vi "Teleop.vi"(10 "Match Info":T1={"Autonomous Elapsed Seconds"=0.0, "TeleOp Elapsed Seconds"=0.0, "Disabled Elapsed Seconds"=0.0, "Visited Autonomous"=FALSE, "Visited TeleOp"=FALSE, "Visited Disabled"=FALSE, "Autonomous Settings"={"Autonomous Style"=enum."Independent", "VI Refnum"=refnum}}, 11 "Call Context":T2) -> ()   [LabVIEW 2015]
doc: "This VI is called for each TeleOp packet received from the DS where the robot is not disabled. It is often used to read from the joysticks and update I/O or to update setpoints for timed control loops. It should complete and return within 20 milliseconds or it may miss DS packets."
uses:
  <vilib>/Rock Robotics/WPI/DriverStation/WPI_DriverStationDerivedRobotMode.ctl
  <vilib>/Rock Robotics/WPI/DriverStation/WPI_DriverStationMatch Info.ctl
  <vilib>/Rock Robotics/Network Tables/NT Read Boolean.vi
  <vilib>/Rock Robotics/Network Tables/NT Read Number.vi
  <vilib>/Rock Robotics/WPI/Utilities/WPI_GetSetVariantRefNum.vi
  <vilib>/Rock Robotics/Network Tables/SD Write Number.vi
  <vilib>/Rock Robotics/Network Tables/SD Write Boolean.vi
panel:
  out "Sample Slider 0":dbl(slide) scale=0.0..5.0
  out "Sample Boolean 1":bool
  out "Sample Boolean 0":bool
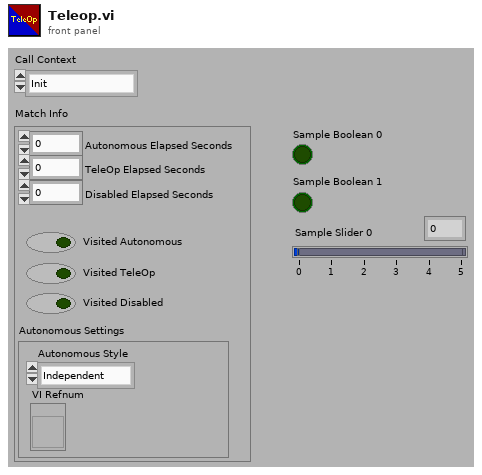
[diagram p1: front panel]
types:
  T1 = typedef "WPI_DriverStationMatch Info.ctl" = cluster{"Autonomous Elapsed Seconds":dbl, "TeleOp Elapsed Seconds":dbl, "Disabled Elapsed Seconds":dbl, "Visited Autonomous":bool, "Visited TeleOp":bool, "Visited Disabled":bool, "Autonomous Settings":cluster{"Autonomous Style":enum16{"Iterative", "Independent"}, "VI Refnum":refnum<vi>}}
  T2 = typedef "WPI_DriverStationDerivedRobotMode.ctl" = enum16{"Init", "Execute", "Stop"}
  T3 = typedef "WPI_JoystickDevRef.ctl" = cluster{"Device":T4}
  T4 = typedef "WPI_JoystickDeviceEnum.ctl" = enum16{"USB 0", "USB 1", "USB 2", "USB 3", "USB 4", "USB 5"}
  T5 = cluster{"Axes[0]":dbl, "Axes[1]":dbl, "Axes[2]":dbl, "Axes[3]":dbl, "Axes[4]":dbl, "Axes[5]":dbl, "Axes[6]":dbl, "Axes[7]":dbl, "Axes[8]":dbl}
  T6 = cluster{"Buttons[0]":bool, "Buttons[1]":bool, "Buttons[2]":bool, "Buttons[3]":bool, "Buttons[4]":bool, "Buttons[5]":bool, "Buttons[6]":bool, "Buttons[7]":bool, "Buttons[8]":bool}
  T7 = typedef "WPI_EncoderDevRef.ctl" = cluster{"DevStatus":errorcluster, "EncoderIndex":T8, "CounterIndex":T9, "DistancePerCount":dbl, "Decoding Type":T10}
  T8 = typedef "FPGA_EncoderIdx.ctl" = enum8{"Enc 0", "Enc 1", "Enc 2", "Enc 3", "Enc 4", "Enc 5", "Enc 6", "Enc 7", "Invalid"}
  T9 = typedef "FPGA_CounterCtrSystemIndex.ctl" = enum8{"Ctr 0", "Ctr 1", "Ctr 2", "Ctr 3", "Ctr 4", "Ctr 5", "Ctr 6", "Ctr 7", "Invalid"}
  T10 = typedef "WPI_EncoderType.ctl" = enum16{"1x", "2x", "4x"}
  T11 = typedef "WPI_RobotDriveDevRef.ctl" = cluster{"DevStatus":errorcluster, "Motors[]":T12[], "Square Inputs":bool, "Max Output":dbl}
  T12 = typedef "WPI_MotorControlDeviceRef.ctl" = cluster{"DeviceStatus":errorcluster, "Type":T13, "PWM":cluster{"PWM Channel":T14, "DeadBand":T15}, "CAN":cluster{"Device Number":u8, "Control Mode":T16, "Semaphore":T17, "Max Vout":dbl, "TalonSRX Control Mode":T18}, "Invert":bool}
  T13 = typedef "WPI_MotorControlType.ctl" = enum16{"PWM", "CAN", "CANTalonSRX"}
  T14 = typedef "FPGA_DIOPWMChannel.ctl" = enum8{"PWM 0", "PWM 1", "PWM 2", "PWM 3", "PWM 4", "PWM 5", "PWM 6", "PWM 7", "PWM 8", "PWM 9", "PWM MXP 0", "PWM MXP 1", "PWM MXP 2", "PWM MXP 3", "PWM MXP 4", "PWM MXP 5", "PWM MXP 6", "PWM MXP 7", "PWM MXP 8", "PWM MXP 9", "Invalid"}
  T15 = typedef "WPI_PWMDeadband.ctl" = cluster{"Name":string, "maxPositivePwm":i32, "minPositivePwm":i32, "centerPwm":i32, "maxNegativePwm":i32, "minNegativePwm":i32, "angularRange":u16}
  T16 = typedef "WPI_CANJaguar_ControlMode.ctl" = enum8{"Percent VBus", "Current", "Speed", "Position", "Voltage"}
  T17 = typedef "Semaphore RefNum" = refnum<k1>
  T18 = typedef "WPI_CANTalonSRX_APIControlMode.ctl" = enum8{"Percent VBus", "Speed", "Position", "Slave", "Unchanged / Invalid", "Voltage Compensation", "Current", "Motion Profile"}
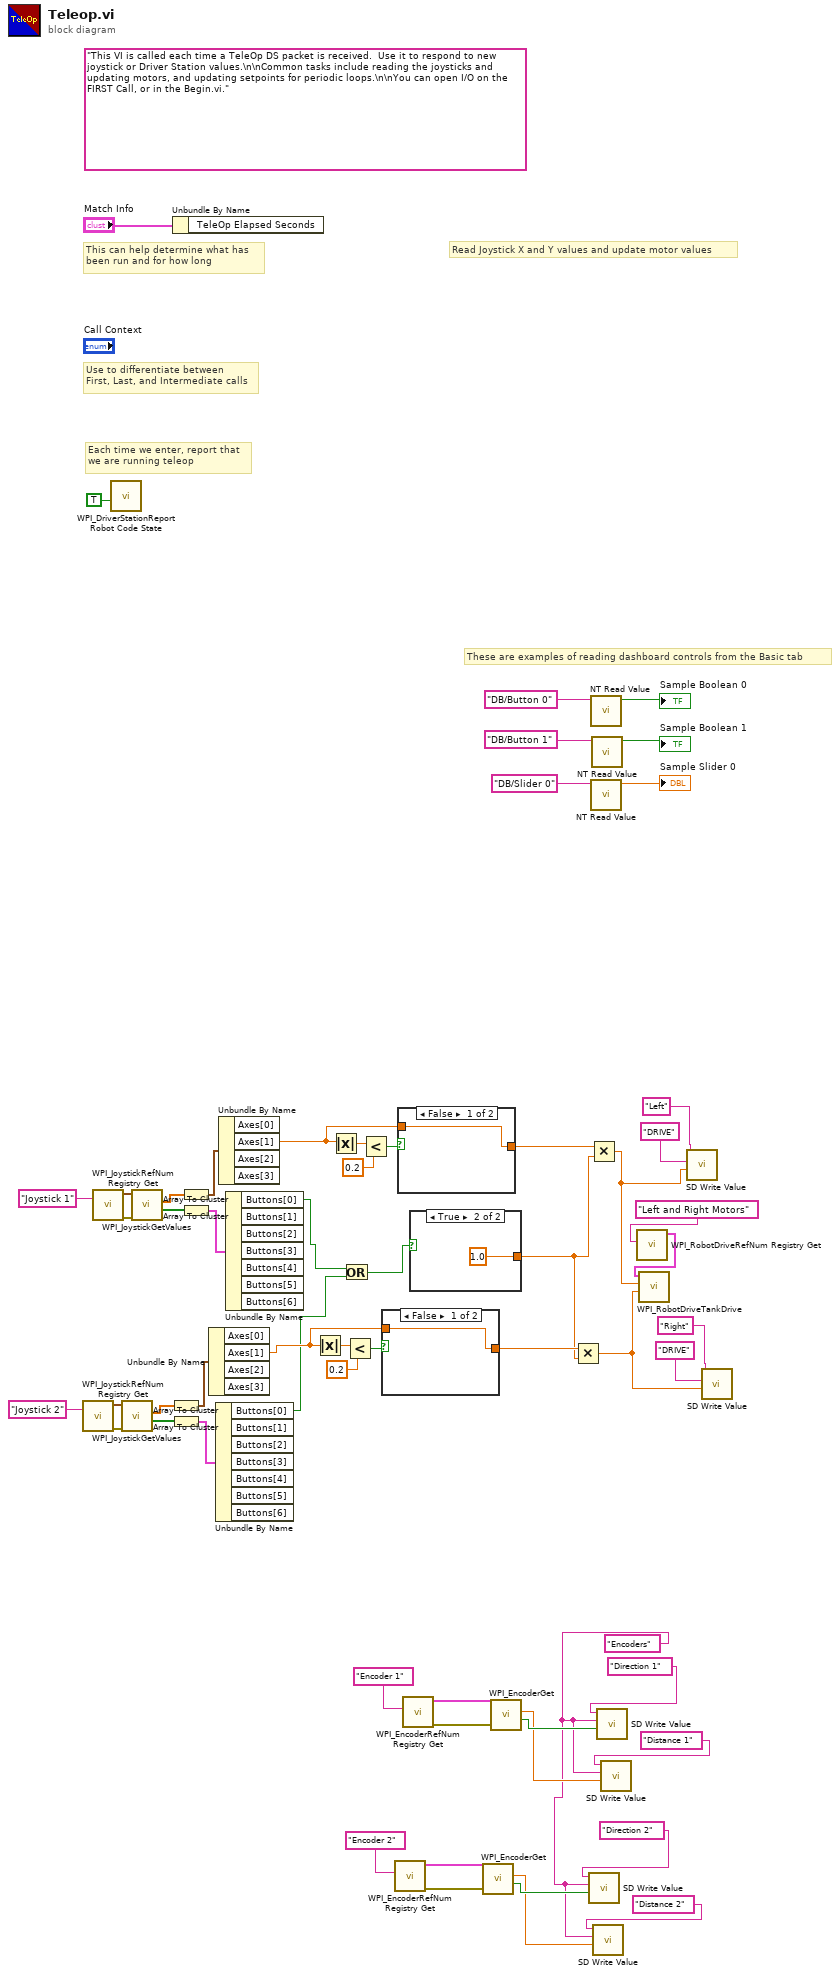
[diagram p0: block diagram]
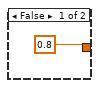
[diagram p2: hidden frame]
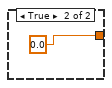
[diagram p3: hidden frame]
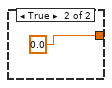
[diagram p4: hidden frame]
diagram:
  w1 = "Encoders"
  (unwired) "This VI is called each time a TeleOp DS packet is received.  Use it to respond to new joystick or Driver Station values.\n\nCommon tasks include reading the joysticks and updating motors, and updating setpoints for periodic loops.\n\nYou can open I/O on the FIRST Call, or in the Begin.vi."
  # "These are examples of reading dashboard controls from the Basic tab"
  # "Each time we enter, report that\nwe are running teleop"
  # "Use to differentiate between\nFirst, Last, and Intermediate calls"
  # "This can help determine what has\nbeen run and for how long"
  # "Read Joystick X and Y values and update motor values"
  n1 = call <vilib>:"WPI_JoystickRefNum Registry Get.vi"("refnum name"="Joystick 2") -> ("error out"=w43:errorcluster, "JoystickDevRef"=w42:T3)  [unwired: 9 in]
  n2 = call <vilib>:"WPI_JoystickRefNum Registry Get.vi"("refnum name"="Joystick 1") -> ("error out"=w50:errorcluster, "JoystickDevRef"=w49:T3)  [unwired: 9 in]
  n3 = call <vilib>:"WPI_DriverStationReport Robot Code State.vi"("TeleOp"=TRUE ("Autonomous")) -> ()  [unwired: 10 in, 1 out]
  n4 = call <vilib>:"WPI_JoystickGetValues.vi"("error in (no error)"=w43, "JoystickDevRef"=w42) -> ("Buttons"=w40:bool[], "Axes"=w41:dbl[])  [unwired: 5 in, 3 out]
  n5 = call <vilib>:"WPI_JoystickGetValues.vi"("error in (no error)"=w50, "JoystickDevRef"=w49) -> ("Buttons"=w47:bool[], "Axes"=w48:dbl[])  [unwired: 5 in, 3 out]
  n6 = Array To Cluster(array=w41) -> (cluster=w39:T5)
  n7 = Array To Cluster(array=w40) -> (cluster=w38:T6)
  n8 = Unbundle By Name("Match Info") -> ()  [unwired: 1 out]
  n9 = Array To Cluster(array=w48) -> (cluster=w46:T5)
  n10 = Array To Cluster(array=w47) -> (cluster=w45:T6)
  n11 = Unbundle By Name(w39) -> ("Axes[1]"=w28:dbl)  [unwired: 3 out]
  n12 = Unbundle By Name(w38) -> ("Buttons[0]"=w17:bool)  [unwired: 6 out]
  n13 = Unbundle By Name(w46) -> ("Axes[1]"=w33:dbl)  [unwired: 3 out]
  n14 = Unbundle By Name(w45) -> ("Buttons[0]"=w18:bool)  [unwired: 6 out]
  n15 = Absolute Value(x=w28) -> (abs(x)=w32:dbl)
  n16 = Absolute Value(x=w33) -> (abs(x)=w37:dbl)
  n17 = Or(x=w18, y=w17) -> (x .or. y?=w16:bool)
  n18 = Less?(x=w32, y=0.2) -> (x < y?=w30:bool)
  n19 = Less?(x=w37, y=0.2) -> (x < y?=w35:bool)
  n20 = case shown="False" w30 {
    tunnel: [w60 0.0] -> w29
    tunnel: w28 -> [w60 _]
    frame False {
    }
    frame True {
    }
  }
  n21 = call <vilib>:"WPI_EncoderRefNum Registry Get.vi"("refnum name"="Encoder 2") -> ("error out"=w7:errorcluster, "EncoderDevRef"=w6:T7)  [unwired: 9 in]
  n22 = case shown="False" w35 {
    tunnel: [w62 0.0] -> w34
    tunnel: w33 -> [w62 _]
    frame False {
    }
    frame True {
    }
  }
  n23 = call <vilib>:"WPI_EncoderRefNum Registry Get.vi"("refnum name"="Encoder 1") -> ("error out"=w14:errorcluster, "EncoderDevRef"=w13:T7)  [unwired: 9 in]
  n24 = case shown="True" w16 {
    tunnel: [0.8 1.0] -> w27
    frame False {
    }
    frame True {
    }
  }
  n25 = call <vilib>:"WPI_EncoderGet.vi"("error in (no error)"=w7, "EncoderDevRef"=w6) -> ("Direction"=w5:bool, "Distance"=w3:dbl)  [unwired: 4 in, 4 out]
  n26 = call <vilib>:"WPI_EncoderGet.vi"("error in (no error)"=w14, "EncoderDevRef"=w13) -> ("Direction"=w12:bool, "Distance"=w10:dbl)  [unwired: 4 in, 4 out]
  n27 = Multiply(x=w29, y=w27) -> (x*y=w22:dbl)
  n28 = Multiply(x=w34, y=w27) -> (x*y=w19:dbl)
  n29 = call-poly <vilib>:"SD Write Value.vi"("Boolean"=w5, "Table Prefix"=w1, "Name"="Direction 2") -> ()  [unwired: 7 in, 2 out]
  n30 = call-poly <vilib>:"NT Read Value.vi"("Name"="DB/Button 0" ("refnum name")) -> ("Boolean"=→"Sample Boolean 0":bool)  [unwired: 9 in, 1 out]
  n31 = call-poly <vilib>:"NT Read Value.vi"("Name"="DB/Slider 0" ("refnum name")) -> ("Numeric"=→"Sample Slider 0":dbl)  [unwired: 9 in, 1 out]
  n32 = call-poly <vilib>:"NT Read Value.vi"("Name"="DB/Button 1" ("refnum name")) -> ("Boolean"=→"Sample Boolean 1":bool)  [unwired: 9 in, 1 out]
  n33 = call-poly <vilib>:"SD Write Value.vi"("Numeric"=w3, "Table Prefix"=w1, "Name"="Distance 2") -> ()  [unwired: 7 in, 2 out]
  n34 = call-poly <vilib>:"SD Write Value.vi"("Boolean"=w12, "Table Prefix"=w1, "Name"="Direction 1") -> ()  [unwired: 7 in, 2 out]
  n35 = call-poly <vilib>:"SD Write Value.vi"("Numeric"=w10, "Table Prefix"=w1, "Name"="Distance 1") -> ()  [unwired: 7 in, 2 out]
  n36 = call <vilib>:"WPI_RobotDriveRefNum Registry Get.vi"("refnum name"="Left and Right Motors") -> ("RobotDriveDevRef"=w26:T11)  [unwired: 9 in, 1 out]
  n37 = call <vilib>:"WPI_RobotDriveTankDrive.vi"("Right axis value"=w22, "Left axis value"=w19, "RobotDriveDevRef"=w26) -> ()  [unwired: 6 in, 3 out]
  n38 = call-poly <vilib>:"SD Write Value.vi"("Numeric"=w19, "Table Prefix"="DRIVE", "Name"="Left") -> ()  [unwired: 7 in, 2 out]
  n39 = call-poly <vilib>:"SD Write Value.vi"("Numeric"=w22, "Table Prefix"="DRIVE", "Name"="Right") -> ()  [unwired: 7 in, 2 out]
